vi "Register gRPC Messages.vi"(8 "error in (no error)":errorcluster, 11 "gRPCid":T1) -> (0 "error out":errorcluster, 3 "gRPCid":T1)   [LabVIEW 2019, in "Discovery_client.lvlib" / "Discovery_client.lvclass"]
uses:
  Discovery_client.lvclass
  <vilib>/gRPC/LabVIEW gRPC Library/Server API/typeDefs/grpcId.ctl
  <vilib>/gRPC/LabVIEW gRPC Library/Server API/typeDefs/Message Metadata.ctl
  <vilib>/gRPC/LabVIEW gRPC Library/Server API/typeDefs/Message Element Metadata.ctl
  <vilib>/gRPC/LabVIEW gRPC Library/Server API/typeDefs/Message Element Type.ctl
  <vilib>/gRPC/LabVIEW gRPC Library/gprc-lvsupport-release.lvlib
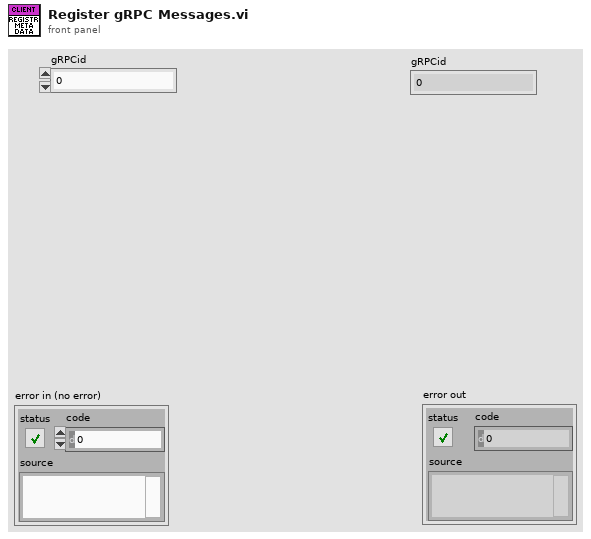
[diagram p1: front panel]
types:
  T1 = typedef "gprc-lvsupport-release.lvlib/grpcId.ctl" = u64
  T2 = typedef "gprc-lvsupport-release.lvlib/Message Metadata.ctl" = cluster{"Version":i32, "Name":string, "Type Url":string, "Elements":T3[]}
  T3 = typedef "gprc-lvsupport-release.lvlib/Message Element Metadata.ctl" = cluster{"Embedded Message Name":string, "Protobuf Index":i32, "MessageElementType":T4, "Repeated":bool}
  T4 = typedef "gprc-lvsupport-release.lvlib/Message Element Type.ctl" = enum32{"Int32Value", "FloatValue", "DoubleValue", "BoolValue", "StringValue", "MessageValue", "Int64Value", "UInt32Value", "UInt64Value", "EnumValue", "Bytes", "Fixed64", "Fixed32", "SFixed64", "SFixed32", "SInt64", "SInt32"}
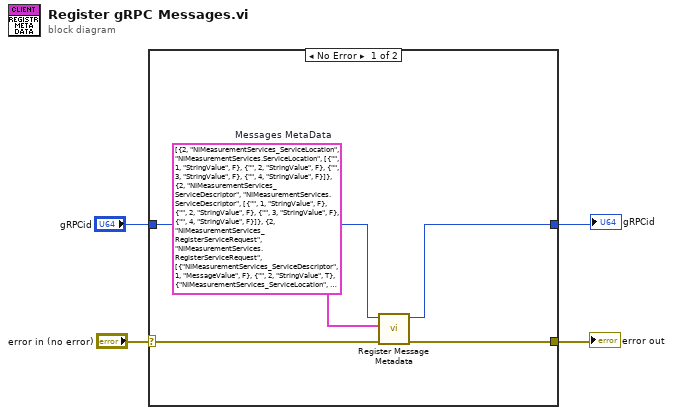
[diagram p0: block diagram]
diagram:
  n1 = case shown="No Error" "error in (no error)" {
    selector: "error in (no error)" -> [w9 w11]
    tunnel: [w8 w11] -> w3
    tunnel: "gRPCid" -> [w7 w10]
    tunnel: [w5 w10] -> w1
    frame No Error {
      w6 = T2[] [{"Version"=2, "Name"="NIMeasurementServices_ServiceLocation", "Type Url"="NIMeasurementServices.ServiceLocation", "Elements"=[{"Embedded Message Name"="", "Protobuf Index"=1, "MessageElementType"=enum."StringValue", "Repeated"=FALSE}, {"Embedded Message Name"="", "Protobuf Index"=2, "MessageElementType"=enum."StringValue", "Repeated"=FALSE}, {"Embedded Message Name"="", "Protobuf Index"=3, "MessageElementType"=enum."StringValue", "Repeated"=FALSE}, {"Embedded Message Name"="", "Protobuf Index"=4, "MessageElementType"=enum."StringValue", "Repeated"=FALSE}]}, {"Version"=2, "Name"="NIMeasurementServices_ServiceDescriptor", "Type Url"="NIMeasurementServices.ServiceDescriptor", "Elements"=[{"Embedded Message Name"="", "Protobuf Index"=1, "MessageElementType"=enum."StringValue", "Repeated"=FALSE}, {"Embedded Message Name"="", "Protobuf Index"=2, "MessageElementType"=enum."StringValue", "Repeated"=FALSE}, {"Embedded Message Name"="", "Protobuf Index"=3, "MessageElementType"=enum."StringValue", "Repeated"=FALSE}, {"Embedded Message Name"="", "Protobuf Index"=4, "MessageElementType"=enum."StringValue", "Repeated"=FALSE}]}, {"Version"=2, "Name"="NIMeasurementServices_RegisterServiceRequest", "Type Url"="NIMeasurementServices.RegisterServiceRequest", "Elements"=[{"Embedded Message Name"="NIMeasurementServices_ServiceDescriptor", "Protobuf Index"=1, "MessageElementType"=enum."MessageValue", "Repeated"=FALSE}, {"Embedded Message Name"="", "Protobuf Index"=2, "MessageElementType"=enum."StringValue", "Repeated"=TRUE}, {"Embedded Message Name"="NIMeasurementServices_ServiceLocation", "Protobuf Index"=3, "MessageElementType"=enum."MessageValue", "Repeated"=FALSE}]}, {"Version"=2, "Name"="NIMeasurementServices_RegisterServiceResponse", "Type Url"="NIMeasurementServices.RegisterServiceResponse", "Elements"=[{"Embedded Message Name"="", "Protobuf Index"=1, "MessageElementType"=enum."StringValue", "Repeated"=FALSE}]}, {"Version"=2, "Name"="NIMeasurementServices_UnregisterServiceRequest", "Type Url"="NIMeasurementServices.UnregisterServiceRequest", "Elements"=[{"Embedded Message Name"="", "Protobuf Index"=1, "MessageElementType"=enum."StringValue", "Repeated"=FALSE}]}, {"Version"=2, "Name"="NIMeasurementServices_UnregisterServiceResponse", "Type Url"="NIMeasurementServices.UnregisterServiceResponse", "Elements"=[]}, {"Version"=2, "Name"="NIMeasurementServices_EnumerateServicesRequest", "Type Url"="NIMeasurementServices.EnumerateServicesRequest", "Elements"=[{"Embedded Message Name"="", "Protobuf Index"=1, "MessageElementType"=enum."StringValue", "Repeated"=FALSE}]}, {"Version"=2, "Name"="NIMeasurementServices_EnumerateServicesResponse", "Type Url"="NIMeasurementServices.EnumerateServicesResponse", "Elements"=[{"Embedded Message Name"="NIMeasurementServices_ServiceDescriptor", "Protobuf Index"=1, "MessageElementType"=enum."MessageValue", "Repeated"=TRUE}]}, {"Version"=2, "Name"="NIMeasurementServices_EnumerateAllServicesRequest", "Type Url"="NIMeasurementServices.EnumerateAllServicesRequest", "Elements"=[]}, {"Version"=2, "Name"="NIMeasurementServices_EnumerateAllServicesResponse", "Type Url"="NIMeasurementServices.EnumerateAllServicesResponse", "Elements"=[{"Embedded Message Name"="NIMeasurementServices_ServiceDescriptor", "Protobuf Index"=1, "MessageElementType"=enum."MessageValue", "Repeated"=TRUE}]}, {"Version"=2, "Name"="NIMeasurementServices_ResolveServiceRequest", "Type Url"="NIMeasurementServices.ResolveServiceRequest", "Elements"=[{"Embedded Message Name"="", "Protobuf Index"=1, "MessageElementType"=enum."StringValue", "Repeated"=FALSE}, {"Embedded Message Name"="", "Protobuf Index"=2, "MessageElementType"=enum."StringValue", "Repeated"=FALSE}]}, {"Version"=2, "Name"="NIMeasurementServices_ResolveMonikerEndpointRequest", "Type Url"="NIMeasurementServices.ResolveMonikerEndpointRequest", "Elements"=[{"Embedded Message Name"="", "Protobuf Index"=1, "MessageElementType"=enum."StringValue", "Repeated"=FALSE}, {"Embedded Message Name"="NIMeasurementServices_ServiceLocation", "Protobuf Index"=2, "MessageElementType"=enum."MessageValue", "Repeated"=FALSE}]}]  # Messages MetaData
      n2 = call <vilib>:"Register Message Metadata.vi"("error in (no error)"=w9, "Messages"=w6, "gRPCid"=w7) -> ("error out"=w8:errorcluster, "gRPCid"=w5:T1)  [unwired: 7 in]
    }
    frame Error {
    }
  }
  "error out" <- w3
  "gRPCid" <- w1
